vi "Test Report Contain TestCase Time.vi"(8 "error in (no error)":errorcluster, 11 "XML Report Test in":refnum<class "XML Report Test.lvclass">) -> (0 "error out":errorcluster, 3 "XML Report Test out":refnum<class "XML Report Test.lvclass">)   [LabVIEW 2020, in "XML Report Test.lvclass"]
uses:
  XML Report Test.lvclass
  XML Report Test.lvclass/XML Report Test.ctl
  source/Plugins/XML Report/XML Report.lvclass
panel:
  out "Report Content":string
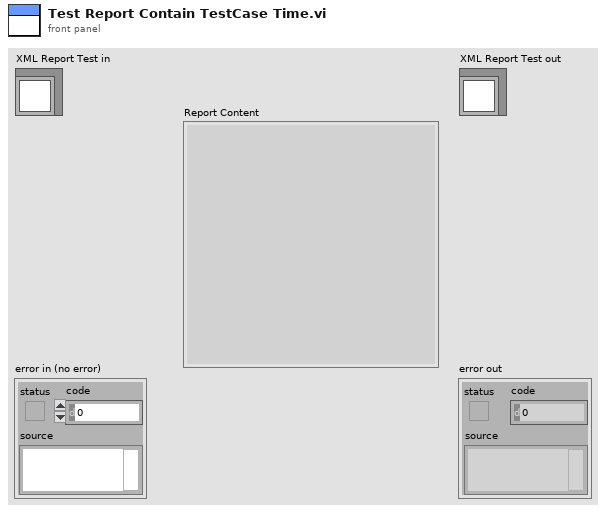
[diagram p1: front panel]
types:
  T1 = typedef "Result.lvlib/Result.ctl" = cluster{"Name":string, "Description":string, "Status":T2, "Result Type":T3, "Execution Time":dbl, "Data":cluster{"Expected":variant, "Actual":variant, "Delta":variant}}
  T2 = typedef "Result.lvlib/Status.ctl" = enum16{"", "Passed", "Failed", "Error", "Skipped", "Setup Error", "Broken", "Teardown Error"}
  T3 = typedef "Result.lvlib/Type.ctl" = enum16{"Test Case", "Test Suite", "Test Run", "Pass", "Fail", "Skip", "Pass if", "Fail if", "Pass if Error", "Fail if Error", "Pass if Equal", "Fail if Equal"}
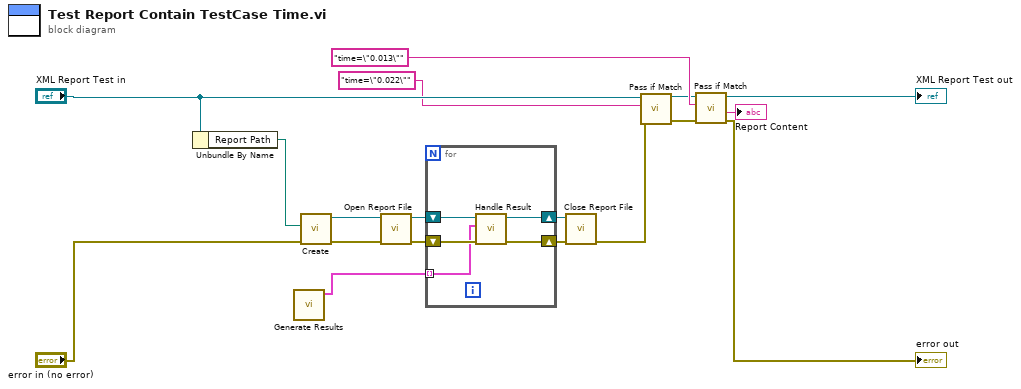
[diagram p0: block diagram]
diagram:
  n1 = Unbundle By Name("XML Report Test in") -> ("Report Path"=w1:path)
  n2 = call "Generate Results.vi"() -> ("Data"=w9:T1[])  [unwired: 10 in, 1 out]
  n3 = call "Create.vi"("error in (no error)"="error in (no error)", "Report Path"=w1) -> ("error out"=w3:errorcluster, "XML Report"=w2:refnum<class "XML Report.lvclass">)  [unwired: 8 in]
  n4 = call-dynamic "Open Report File.vi"("error in (no error)"=w3, "XML Report In"=w2) -> ("error out"=w18:errorcluster, "XML Report Out"=w11:refnum<class "XML Report.lvclass">)  [unwired: 8 in]
  n5 = for {
    shift-right: [w22] -> w12
    shift-left: w18 -> [w23]
    shift-right: [w20] -> w10
    shift-left: w11 -> [w21]
    tunnel: w9 -> [w19] mode=indexing
    n6 = call-dynamic "Handle Result.vi"("error in (no error)"=w23, "Result"=w19, "XML Report In"=w21) -> ("error out"=w22:errorcluster, "XML Report Out"=w20:refnum<class "XML Report.lvclass">)  [unwired: 7 in]
  }
  n7 = call-dynamic "Close Report File.vi"("error in (no error)"=w12, "XML Report In"=w10) -> ("error out"=w15:errorcluster)  [unwired: 8 in, 1 out]
  n8 = call "Pass if Match.vi"("error in (no error)"=w15, "regular expression"="time=\"0.022\"", "XML Report Test in"="XML Report Test in") -> ("error out"=w7:errorcluster, "XML Report Test out"=w6:refnum<class "XML Report Test.lvclass">)  [unwired: 6 in, 1 out]
  n9 = call "Pass if Match.vi"("error in (no error)"=w7, "regular expression"="time=\"0.013\"", "XML Report Test in"=w6) -> ("error out"=→"error out":errorcluster, "Report Content"=→"Report Content":string, "XML Report Test out"=→"XML Report Test out":refnum<class "XML Report Test.lvclass">)  [unwired: 6 in]
